vi "YAFFooter_SendUiEvent.vi"(7 "UiEventNames":T1, 8 "ErrorIn":errorcluster, 9 "Data":variant, 11 "YAFFooter:YAFFooter in":refnum<class "YAFFooter.lvclass">) -> (0 "ErrorOut":errorcluster, 3 "YAFFooter:YAFFooter out":refnum<class "YAFFooter.lvclass">)   [LabVIEW 2021, in "YAFFooter.lvlib" / "YAFFooter.lvclass"]
uses:
  YAFFooter.lvclass
  YAFFooter_UiCallBackEvents.ctl
  YAFFooter.lvclass/YAFFooter.ctl
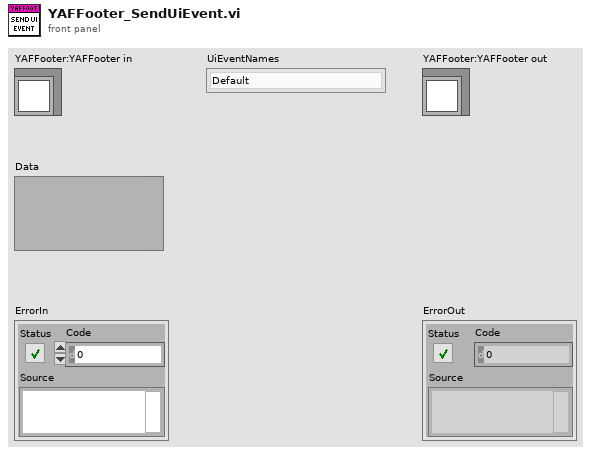
[diagram p1: front panel]
types:
  T1 = typedef "YAFFooter.lvlib/YAFFooter.lvclass/YAFFooter_UiCallBackEvents.ctl" = enum16{"Default", "PersistentDataUpdated"}
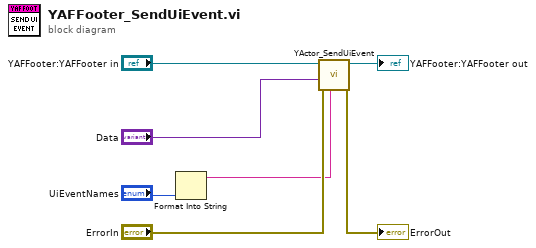
[diagram p0: block diagram]
diagram:
  n1 = Format Into String("UiEventNames") -> (resulting string=w2:string)  [unwired: 3 in, 1 out]
  n2 = call-dynamic "YActor_SendUiEvent.vi"("Event"=w2, "ErrorIn"="ErrorIn", "Data"="Data", "YActorIn"="YAFFooter:YAFFooter in") -> ("ErrorOut"=→"ErrorOut":errorcluster, "YActorOut"=→"YAFFooter:YAFFooter out":refnum<class "YAFFooter.lvclass">)  [unwired: 6 in]
